vi "LvDataToString.vi"(8 "error in (no error)":errorcluster, 11 "Variant":variant) -> (0 "error out":errorcluster, 3 "String Value":string)   [LabVIEW 2015, in "TableLogger_Actor.lvlib" / "TableLogger_Actor.lvclass"]
uses:
  TableLogger_Actor.lvclass
panel:
  # "Connector Pane"
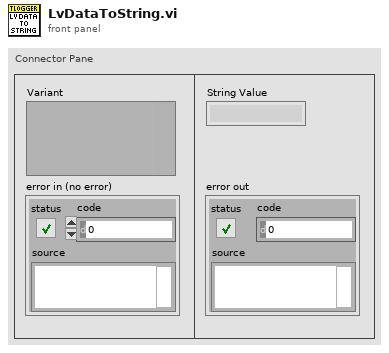
[diagram p1: front panel]
types:
  T1 = typedef "Type Descriptor Enumeration__ogtk.ctl" = enum8{"<Null>", "I8", "I16", "I32", "I64", "U8", "U16", "U32", "U64", "SGL", "DBL", "EXT", "CSG", "CDB", "CXT", "0x0F", "0x10", "0x11", "0x12", "0x13", "0x14", "Enum U8", "Enum U16", "Enum U32", "Enum U64", "SGL PQ", "DBL PQ", "EXT PQ", "CSG PQ", "CDB PQ", "CXT PQ", "0x1F", "0x20", "Boolean", "0x22", "0x23", "0x24", "0x25", "0x26", "0x27", "0x28", "0x29", "0x2A", "0x2B", "0x2C", "0x2D", "0x2E", "0x2F", "String", "0x31", "Path", "Pict", "0x34", "0x35", "0x36", "DAQ", "0x38", "0x39", "0x3A", "0x3B", "0x3C", "0x3D", "0x3E", "0x3F", "Array", "0x41", "0x42", "0x43", "0x44", "0x45", "0x46", "0x47", "0x48", "0x49", "0x4A", "0x4B", "0x4C", "0x4D", "0x4E", "0x4F", "Cluster", "0x51", "0x52", "Variant", "Waveform", "0x55", "0x56", "0x57", "0x58", "0x59", "0x5A", "0x5B", "0x5C", "0x5D", "0x5E", "0x5F", "0x60", "0x61", "0x62", "0x63", "0x64", "0x65", "0x66", "0x67", "0x68", "0x69", "0x6A", "0x6B", "0x6C", "0x6D", "0x6E", "0x6F", "Refnum"}
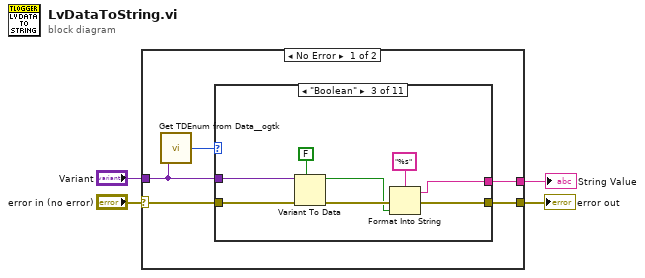
[diagram p0: block diagram]
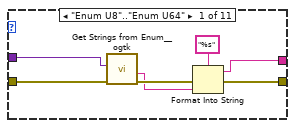
[diagram p2: hidden frame]
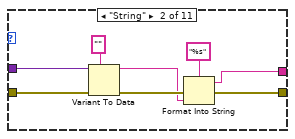
[diagram p3: hidden frame]
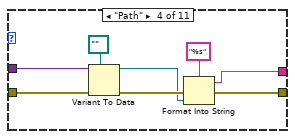
[diagram p4: hidden frame]
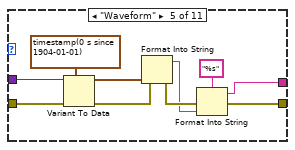
[diagram p5: hidden frame]
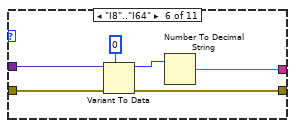
[diagram p6: hidden frame]
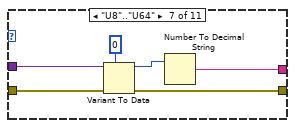
[diagram p7: hidden frame]
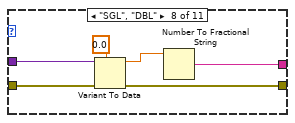
[diagram p8: hidden frame]
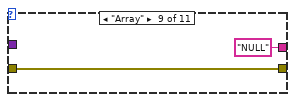
[diagram p9: hidden frame]
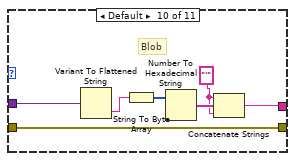
[diagram p10: hidden frame]
diagram:
  n1 = case shown="No Error" "error in (no error)" {
    selector: "error in (no error)" -> [w8 w79]
    tunnel: [w9 w79] -> w4
    tunnel: [w7 _] -> w2
    tunnel: "Variant" -> [w6 _]
    frame No Error {
      n2 = call <userlib>:"Get TDEnum from Data__ogtk.vi"("Data"=w6) -> ("Type Descriptor Enumeration"=w5:T1)  [unwired: 4 in]
      n3 = case shown="\"Boolean\"" w5 {
        tunnel: [w12 w19 w27 w35 w43 w52 w58 w64 "NULL" ("String Value") w73 _] -> w7
        tunnel: w8 -> [w16 w24 w32 w40 w50 w56 w62 w68 w70 w72 w78]
        tunnel: w6 -> [w15 w23 w31 w39 w49 w55 w61 w67 _ w77 _]
        tunnel: [w13 w20 w28 w36 w44 w51 w57 w63 w70 w72 w78] -> w9
        frame "Enum U8".."Enum U64" {
          n4 = call <userlib>:"Get Strings from Enum__ogtk.vi"("error in (no error)"=w16, "Enum"=w15) -> ("error out"=w14:errorcluster, "String Value"=w11:string)  [unwired: 6 in, 2 out]
          n5 = Format Into String(format string="%s", error in=w14, w11) -> (resulting string=w12:string, error out=w13:errorcluster)  [unwired: 1 in]
        }
        frame "String" {
          n6 = Variant To Data(error in=w24, type="", Variant=w23) -> (data=w18:string, error out=w21:errorcluster)
          n7 = Format Into String(format string="%s", error in=w21, w18) -> (resulting string=w19:string, error out=w20:errorcluster)  [unwired: 1 in]
        }
        frame "Boolean" {
          n8 = Variant To Data(error in=w32, type=FALSE, Variant=w31) -> (data=w26:bool, error out=w29:errorcluster)
          n9 = Format Into String(format string="%s", error in=w29, w26) -> (resulting string=w27:string, error out=w28:errorcluster)  [unwired: 1 in]
        }
        frame "Path" {
          n10 = Variant To Data(error in=w40, type=path "", Variant=w39) -> (data=w34:path, error out=w37:errorcluster)
          n11 = Format Into String(format string="%s", error in=w37, w34) -> (resulting string=w35:string, error out=w36:errorcluster)  [unwired: 1 in]
        }
        frame "Waveform" {
          n12 = Variant To Data(error in=w50, type=timestamp(0 s since 1904-01-01), Variant=w49) -> (data=w47:timestamp, error out=w46:errorcluster)
          n13 = Format Into String(error in=w46, w47) -> (resulting string=w42:string, error out=w45:errorcluster)  [unwired: 2 in]
          n14 = Format Into String(format string="%s", error in=w45, w42) -> (resulting string=w43:string, error out=w44:errorcluster)  [unwired: 1 in]
        }
        frame "I8".."I64" {
          n15 = Variant To Data(error in=w56, type=i64 0, Variant=w55) -> (data=w53:i64, error out=w51:errorcluster)
          n16 = Number To Decimal String(number=w53) -> (decimal integer string=w52:string)  [unwired: 1 in]
        }
        frame "U8".."U64" {
          n17 = Variant To Data(error in=w62, type=u64 0, Variant=w61) -> (data=w59:u64, error out=w57:errorcluster)
          n18 = Number To Decimal String(number=w59) -> (decimal integer string=w58:string)  [unwired: 1 in]
        }
        frame "SGL", "DBL" {
          n19 = Variant To Data(error in=w68, type=0.0, Variant=w67) -> (data=w65:dbl, error out=w63:errorcluster)
          n20 = Number To Fractional String(number=w65) -> (F-format string=w64:string)  [unwired: 3 in]
        }
        frame "Array" {
        }
        frame Default {
          w71 = "'"
          # "Blob"
          n21 = Variant To Flattened String(Variant=w77) -> (data string=w76:string)  [unwired: 1 out]
          n22 = String To Byte Array(string=w76) -> (unsigned byte array=w75:u8[])
          n23 = Number To Hexadecimal String(2:w75) -> (0:w74:string[])  [unwired: 1 in]
          n24 = Concatenate Strings(w71, w74, w71) -> (w73:string)
        }
        frame "Cluster" {
        }
      }
    }
    frame Error {
    }
  }
  "error out" <- w4
  "String Value" <- w2
